vi "TCP-IP.vi"(6 "Port":i32, 9 "IP Adress":string, 10 "String":string, 11 "Numeric":i32) -> (3 "data out":string)   [LabVIEW 2019]
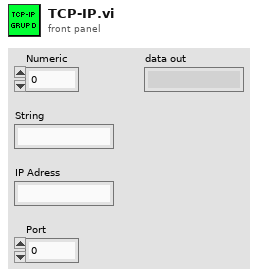
[diagram p1: front panel]
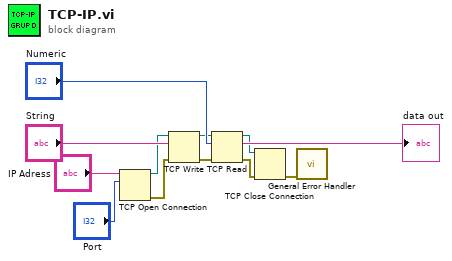
[diagram p0: block diagram]
diagram:
  n1 = TCP Open Connection(address="IP Adress", remote port or service name="Port") -> (connection ID=w3:refnum<k5>, error out=w6:errorcluster)  [unwired: 3 in]
  n2 = TCP Write(connection ID=w3, data in="String", error in (no error)=w6) -> (connection ID out=w2:refnum<k5>, error out=w7:errorcluster)  [unwired: 1 in, 1 out]
  n3 = TCP Read(connection ID=w2, bytes to read="Numeric", error in (no error)=w7) -> (connection ID out=w1:refnum<k5>, data out=→"data out":string, error out=w8:errorcluster)  [unwired: 2 in]
  n4 = TCP Close Connection(connection ID=w1, error in (no error)=w8) -> (error out=w9:errorcluster)  [unwired: 1 in, 1 out]
  n5 = call <vilib>:"General Error Handler.vi"("error in (no error)"=w9) -> ()  [unwired: 10 in, 5 out]
